vi "nirviControlTypeTemplate.vi"() -> ()   [LabVIEW 2017]
panel:
  in  "TF[]":bool[](array[boolean])
  in  "TF":bool
  in  "U8":u8
  in  "U16":u16
  in  "U32":u32
  in  "I8":i8
  in  "I16":i16
  in  "I32":i32
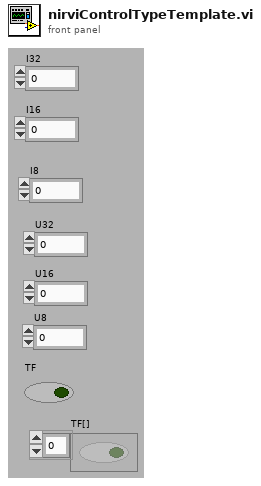
[diagram p1: front panel]
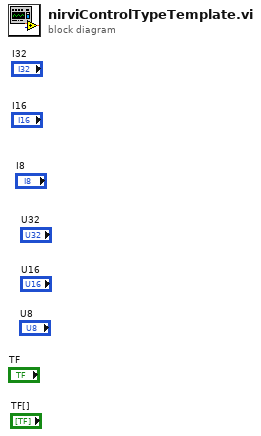
[diagram p0: block diagram]
diagram:
